vi "Control loop.vi"(8 "error in (no error)":errorcluster) -> ()   [LabVIEW 2011]
uses:
  point.ctl
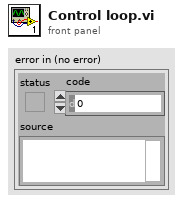
[diagram p1: front panel]
types:
  T1 = enum16{"Startup", "Manual", "Run program", "Home", "Hold position", "Stop"}
  T2 = typedef "point.ctl" = cluster{"X":dbl, "Y":dbl, "Z":dbl, "Ramp":dbl, "Speed":dbl}
  T3 = typedef "WPI_DriverStationRobotMode.ctl" = enum16{"Autonomous Disabled", "Autonomous Enabled", "Teleop Disabled", "Teleop Enabled", "Timeout", "Finish"}
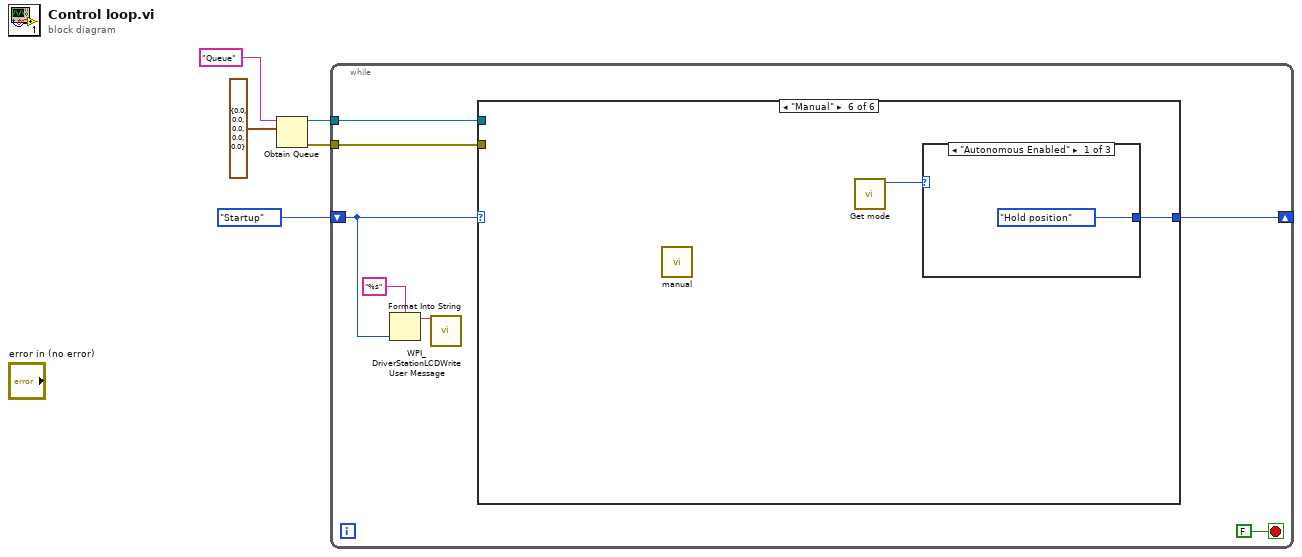
[diagram p0: block diagram]
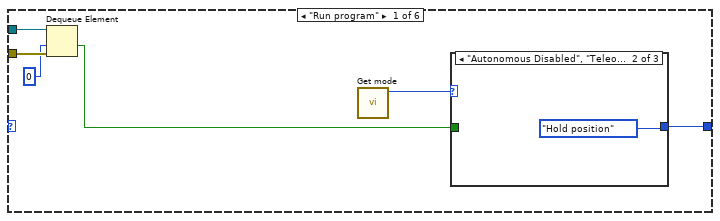
[diagram p2: hidden frame]
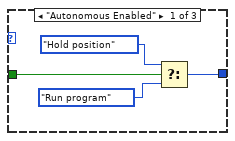
[diagram p3: hidden frame]
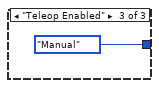
[diagram p4: hidden frame]
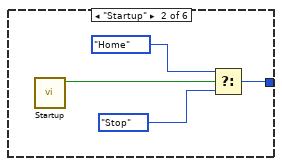
[diagram p5: hidden frame]
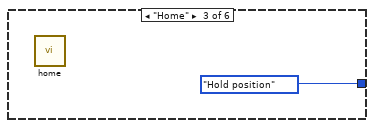
[diagram p6: hidden frame]
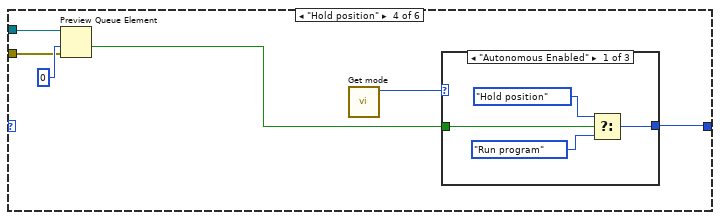
[diagram p7: hidden frame]
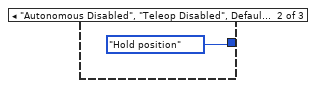
[diagram p8: hidden frame]
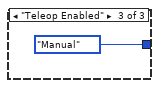
[diagram p9: hidden frame]
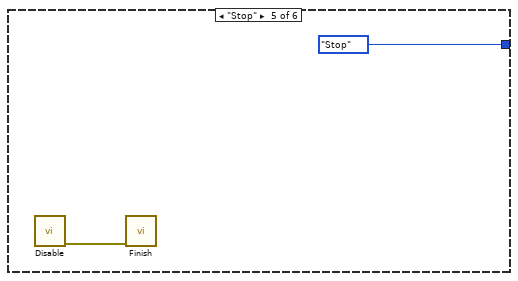
[diagram p10: hidden frame]
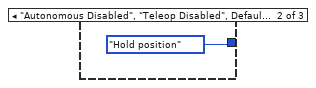
[diagram p11: hidden frame]
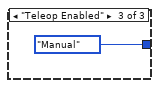
[diagram p12: hidden frame]
diagram:
  n1 = Obtain Queue(name (unnamed)="Queue", element data type=T2 {"X"=0.0, "Y"=0.0, "Z"=0.0, "Ramp"=0.0, "Speed"=0.0} ("Point")) -> (queue out=w5:refnum<queue>, error out=w4:errorcluster)  [unwired: 3 in, 1 out]
  n2 = while {
    shift-right: [w11] -> _
    shift-left: T1."Startup" ("Enum") -> [w6]
    tunnel: w5 -> [w8]
    tunnel: w4 -> [w7]
    stop <- FALSE stop-if-true
    n3 = Format Into String(format string="%s", w6) -> (resulting string=w9:string)  [unwired: 2 in, 1 out]
    n4 = call <vilib>:"WPI_DriverStationLCDWrite User Message.vi"("line text"=w9) -> ()  [unwired: 14 in, 1 out]
    n5 = case shown="\"Manual\"" w6 {
      tunnel: [w14 w27 T1."Hold position" ("Enum") w30 T1."Stop" ("Enum") w44] -> w11
      tunnel: w8 -> [w18 _ _ w34 _ _]
      tunnel: w7 -> [w17 _ _ w33 _ _]
      frame "Run program" {
        n6 = Dequeue Element(queue=w18, timeout in ms (-1)=0, error in (no error)=w17) -> (timed out?=w13:bool)  [unwired: 3 out]
        n7 = call "Get mode.vi"() -> ("Robot Mode"=w15:T3)  [unwired: 11 in]
        n8 = case shown="\"Autonomous Disabled\", \"Teleop Disabled\", Default" w15 {
          tunnel: [w22 T1."Hold position" ("Enum") T1."Manual" ("Enum")] -> w14
          tunnel: w13 -> [w21 _ _]
          frame "Autonomous Enabled" {
            n9 = Select(t=T1."Hold position" ("Enum"), s=w21, f=T1."Run program" ("Enum")) -> (s? t:f=w22:T1)
          }
          frame "Autonomous Disabled", "Teleop Disabled", Default {
          }
          frame "Teleop Enabled" {
          }
        }
      }
      frame "Startup" {
        n10 = call "Startup.vi"() -> ("Good"=w28:bool)  [unwired: 11 in]
        n11 = Select(t=T1."Home" ("Enum"), s=w28, f=T1."Stop" ("Enum")) -> (s? t:f=w27:T1)
      }
      frame "Home" {
        n12 = call "home.vi"() -> ()  [unwired: 12 in]
      }
      frame "Hold position" {
        n13 = Preview Queue Element(queue=w34, timeout in ms (-1)=0, error in (no error)=w33) -> (timed out?=w31:bool)  [unwired: 3 out]
        n14 = call "Get mode.vi"() -> ("Robot Mode"=w32:T3)  [unwired: 11 in]
        n15 = case shown="\"Autonomous Enabled\"" w32 {
          tunnel: [w39 T1."Hold position" ("Enum") T1."Manual" ("Enum")] -> w30
          tunnel: w31 -> [w38 _ _]
          frame "Autonomous Enabled" {
            n16 = Select(t=T1."Hold position" ("Enum"), s=w38, f=T1."Run program" ("Enum")) -> (s? t:f=w39:T1)
          }
          frame "Autonomous Disabled", "Teleop Disabled", Default {
          }
          frame "Teleop Enabled" {
          }
        }
      }
      frame "Stop" {
        n17 = call "Disable.vi"() -> ("error out"=w43:errorcluster)  [unwired: 11 in]
        n18 = call "Finish.vi"("error in (no error)"=w43) -> ()  [unwired: 10 in, 1 out]
      }
      frame "Manual" {
        n19 = call "manual.vi"() -> ()  [unwired: 11 in, 1 out]
        n20 = call "Get mode.vi"() -> ("Robot Mode"=w45:T3)  [unwired: 11 in]
        n21 = case shown="\"Autonomous Enabled\"" w45 {
          tunnel: [T1."Hold position" ("Enum") T1."Hold position" ("Enum") T1."Manual" ("Enum")] -> w44
          frame "Autonomous Enabled" {
          }
          frame "Autonomous Disabled", "Teleop Disabled", Default {
          }
          frame "Teleop Enabled" {
          }
        }
      }
    }
  }
